vi "Dark Current Test All Files For Experiments.vi"() -> ()   [LabVIEW 2020]
uses:
  <instrlib>/CAEN PSM/CAEN PSM.lvlib
panel:
  out "Test is Running 2":bool
  in  "Begin Test 2":bool
  out "7 2":bool
  out "6 2":bool
  out "8 2":bool
  out "5 2":bool
  out "4 2":bool
  out "3 2":bool
  out "2 2":bool
  out "1 2":bool
  out "OVV? 4":bool=TRUE
  out "OVC? 4":bool=TRUE
  out "Actual Voltage Level (V) 4":dbl format="%#_13g"
  out "Actual Current Limit (nA) 2":dbl format="%#_13g"
  in  "dt (s) 2":i32
  out "Time Left (s) 2":dbl
  out "Power Supply Trip 2":bool
  in  "VISA resource name 3":refnum<visa-resource-name>
  in  "Channel # 2":i32
  out "Manual Measurments \nNeeded 2":bool
  in  "Barcodes 2":string[](array[string])
  out "OVV? 3":bool=TRUE
  out "OVC? 3":bool=TRUE
  out "Actual Voltage Level (V) 3":dbl format="%#_13g"
  out "Recorded Current\nfor Previous Tube 2":dbl format="%#_13g"
  in  "Measure Next Tube 2":bool
  out "Next Measurment 2":string
  in  "N 2":i32
  in  "VISA resource name 2":refnum<visa-resource-name>
  in  "Channel #":i32
  out "Power Supply Trip":bool
  out "Time Left (s)":dbl
  out "8":bool
  out "7":bool
  out "6":bool
  out "5":bool
  out "4":bool
  out "3":bool
  out "2":bool
  out "1":bool
  out "Test is Running":bool
  in  "Begin Test":bool
  out "Manual Measurments \nNeeded":bool
  out "OVV? 2":bool=TRUE
  out "OVC? 2":bool=TRUE
  out "Actual Voltage Level (V) 2":dbl format="%#_13g"
  out "Recorded Current\nfor Previous Tube":dbl format="%#_13g"
  in  "Measure Next Tube":bool
  in  "Barcodes":string[](array[string])
  out "Next Measurment":string
  in  "N":i32
  in  "dt (s)":i32
  out "Actual Current Limit (nA)":dbl format="%#_13g"
  out "Actual Voltage Level (V)":dbl format="%#_13g"
  out "OVC?":bool=TRUE
  out "OVV?":bool=TRUE
  # "Dark Current Test"
  # "Instructions in Brief:\n1. Begin the program by clicking the white arrow.\n2. Assemble tubes into the test bench.\n3. Select COM5 for the \"VISA resource name\".\n4. Enter in how often you want to take measurement in the \"dt\" box (typically 60s)\n5. Enter in how many measurments you want to take (typically 15)\n6. Scan in the 8 tubes that you are testing.\n(If you take 15 measurments every 60s, the test will take 15 min.)\n7. Click \"Begin Test\". The \"Test is Running\" LED should light up.\n8. After the intial test, if the total current is below 16nA, \n    the program will write the \n     file and end the test.\n9. If the total current is above 16nA, manual\n    measurments need to be taken.\n10. Engage only the tube indicated by \"Next Measurment\". \n11. Click \"Measure\".\n12. Engage the next tube and continue untill all have been measured.\n13. In both cases, the program will write files and end the test. \n14. The test is over when the \"Test is Running\" LED has turned off."
  # "Green lights indicate tubes that have passed."
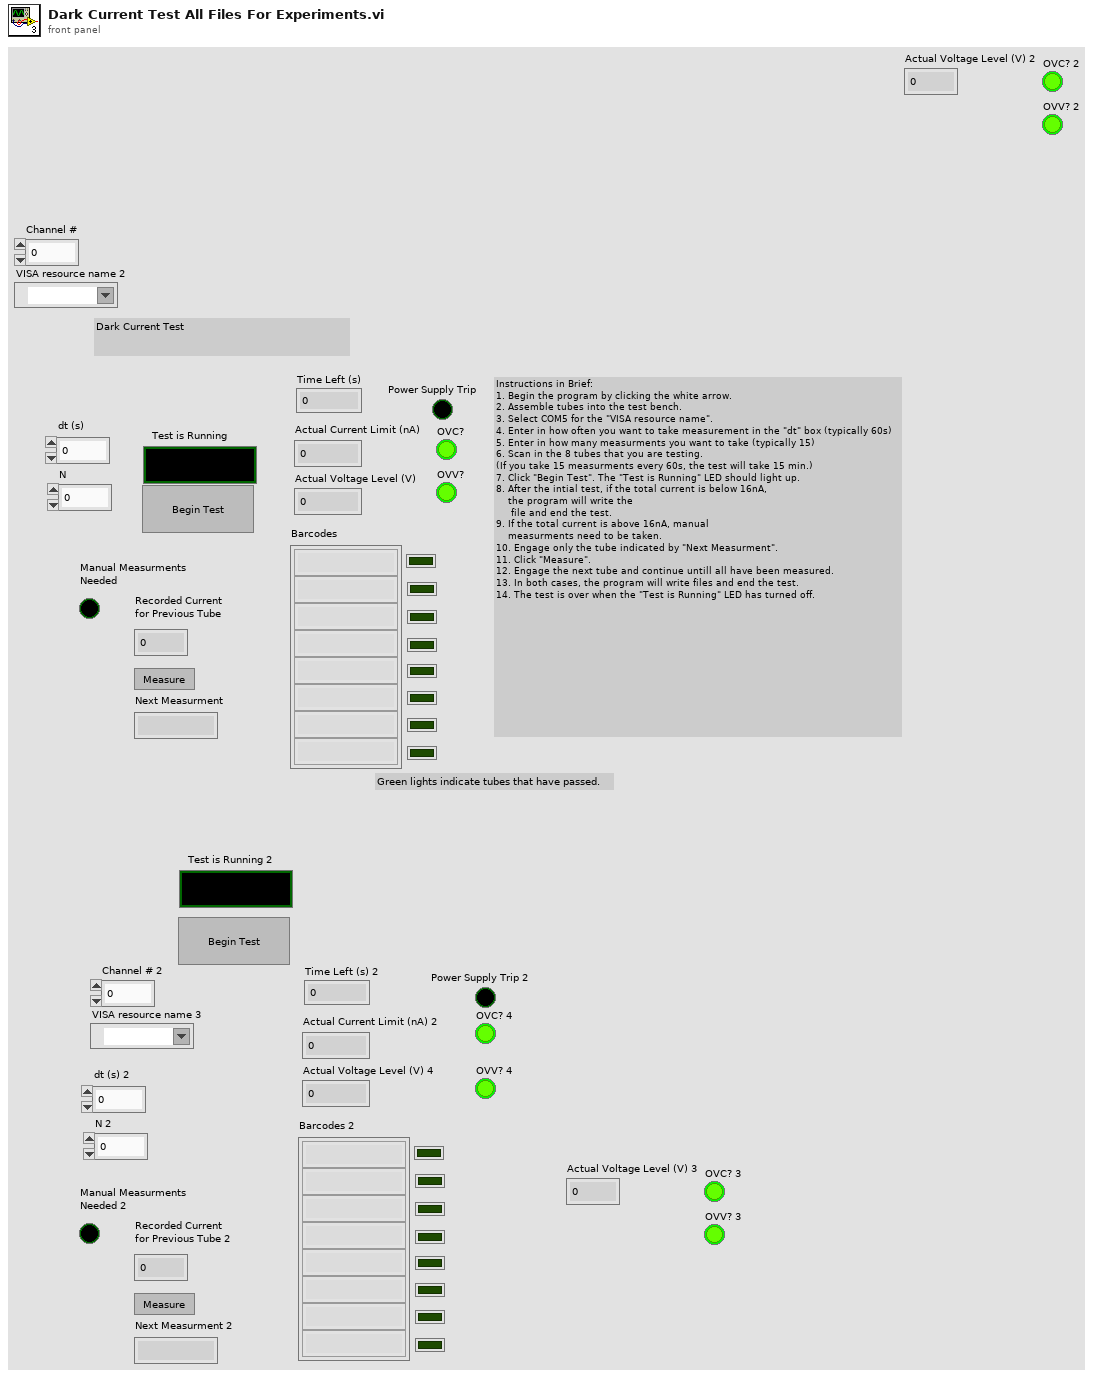
[diagram p1: front panel]
types:
  T1 = cluster{"VISA resource name":refnum<visa-resource-name>, "Board address":u8, "NChannels":u8}
  T2 = cluster{"ON":bool, "RUP":bool, "RDW":bool, "OVC":bool, "OVV":bool, "UNV":bool, "MAXV":bool, "TRIP":bool, "OVP":bool, "OVT":bool, "DIS":bool, "KILL":bool, "ILK":bool, "NOCAL":bool}[]
  T3 = cluster{"ON":bool, "RUP":bool, "RDW":bool, "OVC":bool, "OVV":bool, "UNV":bool, "MAXV":bool, "TRIP":bool, "OVP":bool, "OVT":bool, "DIS":bool, "KILL":bool, "ILK":bool, "NOCAL":bool}
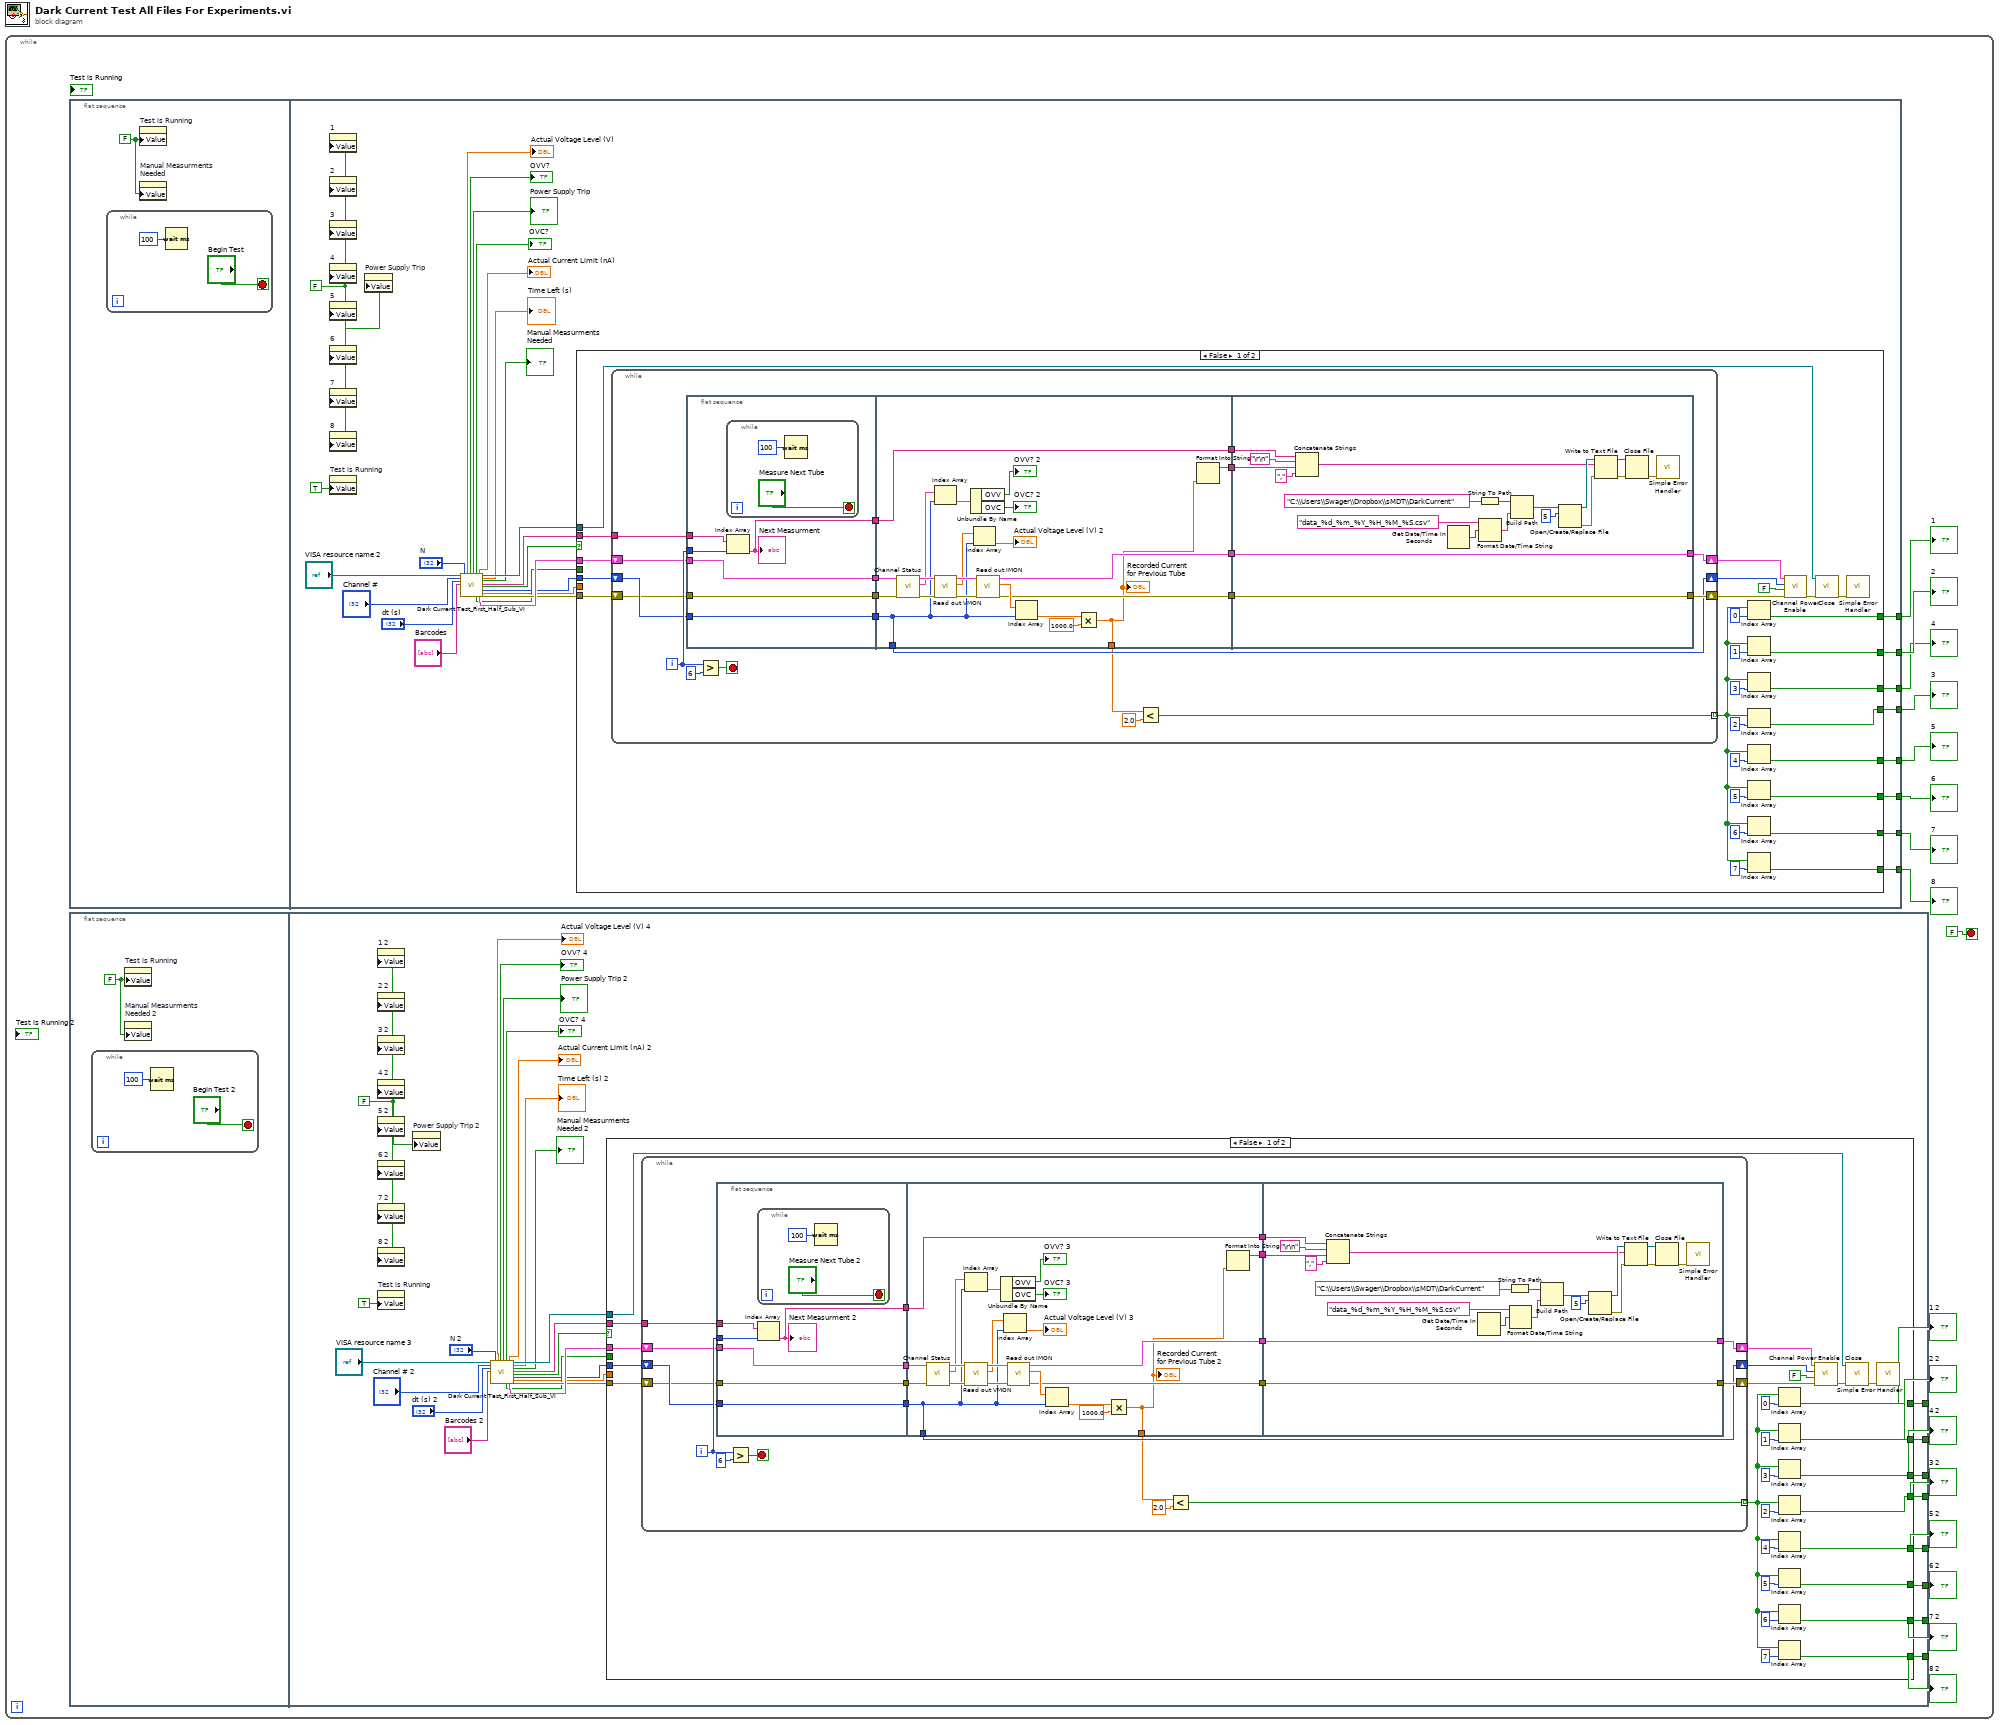
[diagram p0: block diagram]
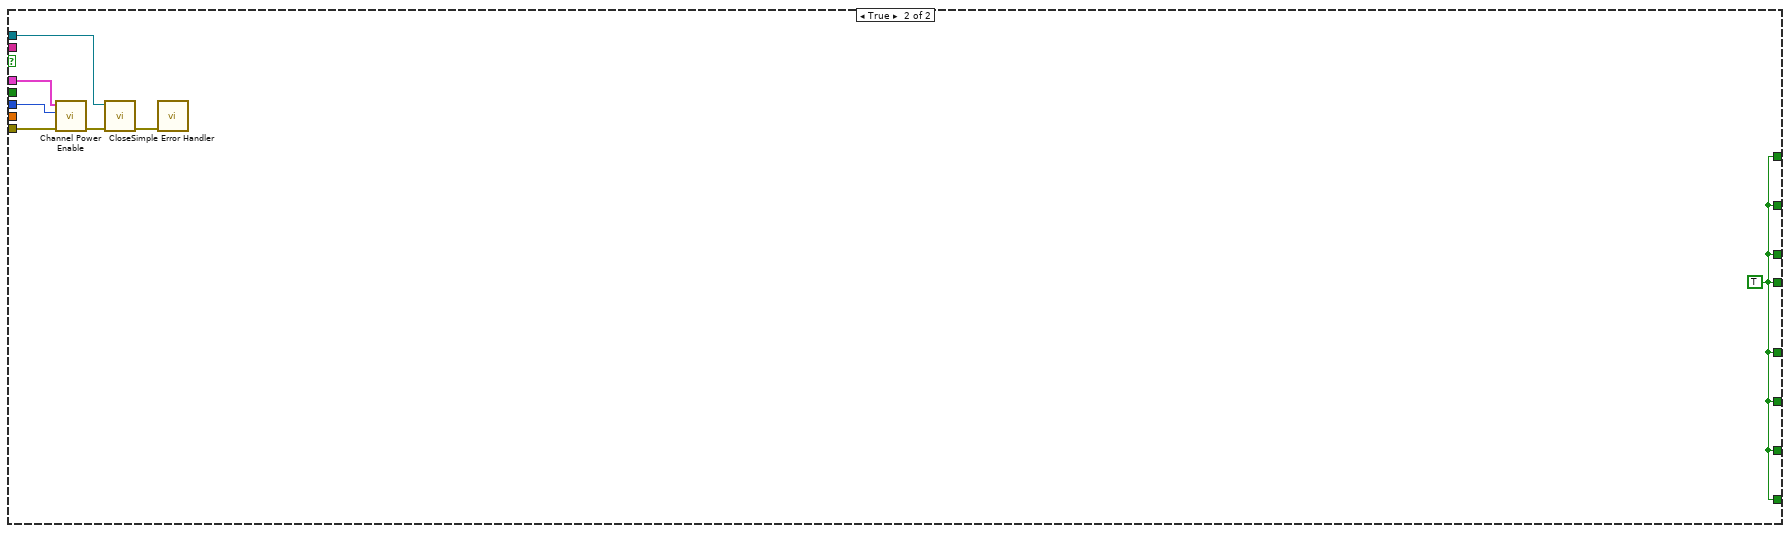
[diagram p2: hidden frame]
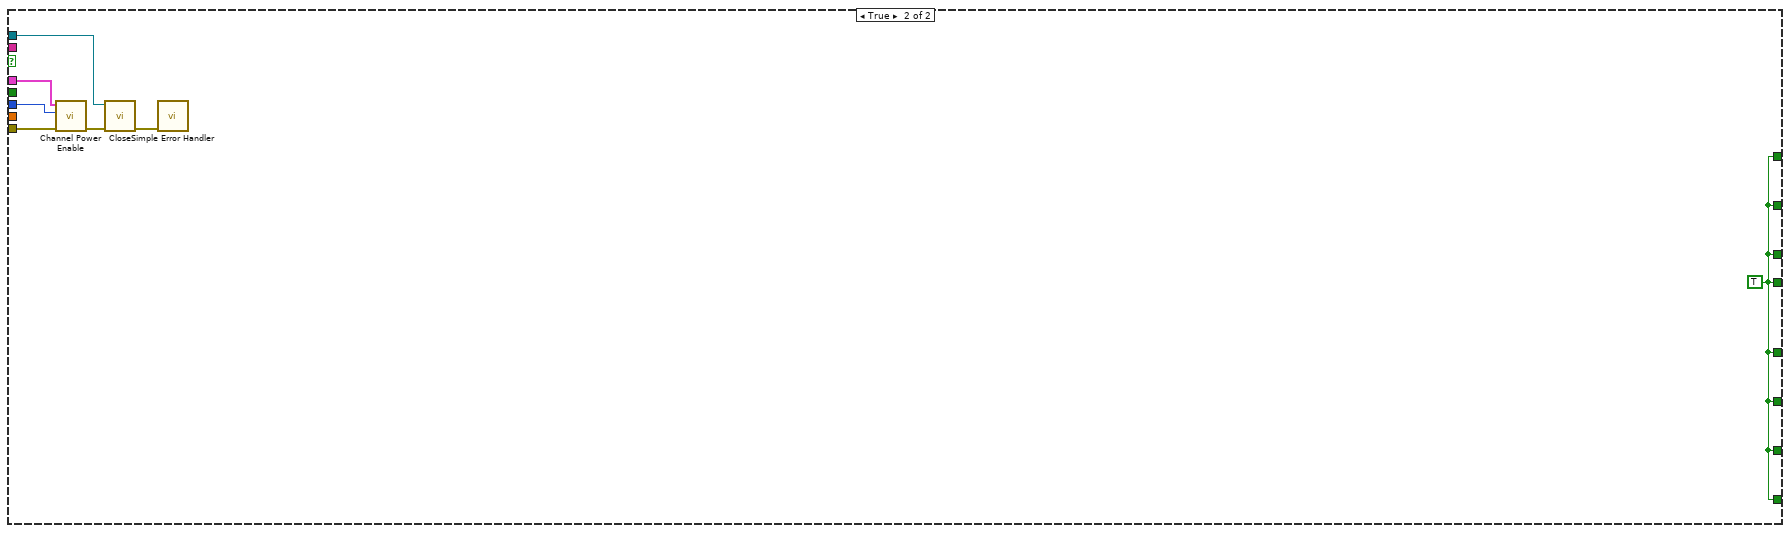
[diagram p3: hidden frame]
diagram:
  n1 = while {
    stop <- FALSE stop-if-true
    n2 = flat-sequence {
      tunnel: [w181] -> w16
      tunnel: [w180] -> w15
      tunnel: [w179] -> w14
      tunnel: [w178] -> w13
      tunnel: [w177] -> w12
      tunnel: [w176] -> w11
      tunnel: [w175] -> w10
      tunnel: [w174] -> w9
      frame #0 {
        w155 = FALSE
        n3 = while {
          stop <- "Begin Test" stop-if-true
          n4 = Wait (ms)(milliseconds to wait=100) -> ()  [unwired: 1 out]
        }
        n5 = property on="Test is Running" class="Bool (strict)"("Value"=w155) -> ()  [unwired: 2 in, 2 out]
        n6 = property on="Manual Measurments \nNeeded" class="Bool (strict)"("Value"=w155) -> ()  [unwired: 2 in, 2 out]
      }
      frame #1 {
        w159 = FALSE
        n7 = property on="1" class="Bool (strict)"("Value"=w159) -> ()  [unwired: 2 in, 2 out]
        n8 = property on="2" class="Bool (strict)"("Value"=w159) -> ()  [unwired: 2 in, 2 out]
        n9 = property on="3" class="Bool (strict)"("Value"=w159) -> ()  [unwired: 2 in, 2 out]
        n10 = property on="4" class="Bool (strict)"("Value"=w159) -> ()  [unwired: 2 in, 2 out]
        n11 = property on="5" class="Bool (strict)"("Value"=w159) -> ()  [unwired: 2 in, 2 out]
        n12 = property on="6" class="Bool (strict)"("Value"=w159) -> ()  [unwired: 2 in, 2 out]
        n13 = property on="7" class="Bool (strict)"("Value"=w159) -> ()  [unwired: 2 in, 2 out]
        n14 = property on="8" class="Bool (strict)"("Value"=w159) -> ()  [unwired: 2 in, 2 out]
        n15 = property on="Test is Running" class="Bool (strict)"("Value"=TRUE) -> ()  [unwired: 2 in, 2 out]
        n16 = property on="Power Supply Trip" class="Bool (strict)"("Value"=w159) -> ()  [unwired: 2 in, 2 out]
        n17 = call "Dark Current Test_First_Half_Sub_VI.vi"("VISA Refnum in"="VISA resource name 2", "Channel #"="Channel #", "dt (s)"="dt (s)", "Barcodes in"="Barcodes", "N"="N") -> ("Actual Voltage Level (V)"=→"Actual Voltage Level (V)":dbl, "OVV?"=→"OVV?":bool, "Power Supply Trip"=→"Power Supply Trip":bool, "OVC?"=→"OVC?":bool, "Boolean 2"=w184:bool, "Actual Current Limit (nA)"=→"Actual Current Limit (nA)":dbl, "BoardHandle out 2"=w186:T1, "VISA Refnum out"=w170:refnum<visa-resource-name>, "Time Left (s)"=→"Time Left (s)":dbl, "Manual Measurments \nNeeded"=→"Manual Measurments \nNeeded":bool, "Barcodes out"=w172:string[], "Boolean"=w182:bool, "Channel # 3"=w183:i32, "Array"=w173:dbl[], "error out"=w185:errorcluster)  [unwired: 8 in]
        n18 = case shown="False" w182 {
          tunnel: w186 -> [w214 w287]
          tunnel: w185 -> [w215 w286]
          tunnel: w184 -> [_ _]
          tunnel: w183 -> [w213 w285]
          tunnel: w170 -> [w209 w288]
          tunnel: w173 -> [_ _]
          tunnel: w172 -> [w205 _]
          tunnel: [w195 w291] -> w181
          tunnel: [w194 w291] -> w180
          tunnel: [w193 w291] -> w179
          tunnel: [w192 w291] -> w178
          tunnel: [w191 w291] -> w177
          tunnel: [w190 w291] -> w176
          tunnel: [w189 w291] -> w175
          tunnel: [w188 w291] -> w174
          frame False {
            n19 = while {
              shift-right: [w221] -> w206
              shift-left: w213 -> [w231]
              shift-right: [w223] -> w208
              shift-left: w214 -> [w228]
              shift-right: [w222] -> w207
              shift-left: w215 -> [w226]
              tunnel: w205 -> [w219]
              tunnel: [w216] -> w204 mode=indexing
              i -> [w234]
              stop <- w235 stop-if-true
              n20 = flat-sequence {
                tunnel: w234 -> [w242]
                tunnel: [w241] -> w233
                tunnel: w231 -> [w240]
                tunnel: [w240] -> w230
                tunnel: [w239] -> w229
                tunnel: w228 -> [w239]
                tunnel: [w238] -> w227
                tunnel: w226 -> [w238]
                tunnel: w219 -> [w237]
                tunnel: w233 -> [w252]
                tunnel: [w252] -> w232
                tunnel: w230 -> [w247]
                tunnel: w229 -> [w250]
                tunnel: w227 -> [w251]
                tunnel: [w249] -> w225
                tunnel: [w248] -> w224
                tunnel: [w247] -> w221
                tunnel: [w246] -> w220
                tunnel: [w245] -> w218
                tunnel: w232 -> [w270]
                tunnel: w225 -> [w268]
                tunnel: w224 -> [w267]
                tunnel: [w268] -> w223
                tunnel: [w267] -> w222
                tunnel: w220 -> [w266]
                frame #0 {
                  n21 = while {
                    stop <- "Measure Next Tube" stop-if-true
                    n22 = Wait (ms)(milliseconds to wait=100) -> ()  [unwired: 1 out]
                  }
                  n23 = Index Array(array=w237, index=w242) -> (element=w241:string)
                  "Next Measurment" <- w241
                }
                frame #1 {
                  n24 = call <instrlib>:"Channel Status.vi"("error in (no error)"=w251, "BoardHandle"=w250) -> ("error out"=w258:errorcluster, "Channel Status Array"=w254:T2, "BoardHandle out"=w259:T1)  [unwired: 7 in]
                  n25 = Index Array(array=w254, index=w247) -> (element=w255:T3)
                  n26 = call <instrlib>:"Read out VMON.vi"("error in (no error)"=w258, "BoardHandle"=w259) -> ("error out"=w262:errorcluster, "VMon values (V)"=w260:dbl[], "BoardHandle out"=w261:T1)  [unwired: 7 in]
                  n27 = Unbundle By Name(w255) -> ("OVV"=→"OVV? 2":bool, "OVC"=→"OVC? 2":bool)
                  n28 = Index Array(array=w260, index=w247) -> (element=→"Actual Voltage Level (V) 2":dbl)
                  n29 = call <instrlib>:"Read out IMON.vi"("error in (no error)"=w262, "BoardHandle"=w261) -> ("error out"=w248:errorcluster, "IMon values (uA)"=w265:dbl[], "BoardHandle out"=w249:T1)  [unwired: 6 in, 1 out]
                  n30 = Index Array(array=w265, index=w247) -> (element=w263:dbl)
                  n31 = Multiply(x=w263, y=1000.0) -> (x*y=w245:dbl)
                  "Recorded Current\nfor Previous Tube" <- w245
                  n32 = Format Into String(w245) -> (resulting string=w246:string)  [unwired: 3 in, 1 out]
                }
                frame #2 {
                  n33 = Concatenate Strings(w270, "\r\n", w266, ",") -> (w272:string)
                  n34 = Get Date/Time In Seconds() -> (seconds since 1Jan1904=w282:timestamp)
                  n35 = String To Path(string="C:\\Users\\Swager\\Dropbox\\sMDT\\DarkCurrent") -> (path=w281:path)
                  n36 = Format Date/Time String(time format string (%c)="data_%d_%m_%Y_%H_%M_%S.csv", seconds (now)=w282) -> (date/time string=w283:string)  [unwired: 1 in]
                  n37 = Build Path(base path=w281, name or relative path=w283) -> (appended path=w279:path)
                  n38 = Open/Create/Replace File(file path (use dialog)=w279, operation (0:open)=5) -> (refnum out=w278:refnum<file>, error out=w277:errorcluster)  [unwired: 4 in, 1 out]
                  n39 = Write to Text File(file (use dialog)=w278, text=w272, error in=w277) -> (refnum out=w276:refnum<file>, error out=w275:errorcluster)  [unwired: 1 in, 1 out]
                  n40 = Close File(refnum=w276, error in=w275) -> (error out=w274:errorcluster)  [unwired: 1 out]
                  n41 = call <vilib>:"Simple Error Handler.vi"("error in (no error)"=w274) -> ()  [unwired: 4 in, 5 out]
                }
              }
              n42 = Greater?(x=w234, y=6) -> (0:w235:bool)
              n43 = Less?(x=w218, y=2.0) -> (x < y?=w216:bool)
            }
            n44 = Index Array(array=w204, index=0) -> (element=w195:bool)
            n45 = Index Array(array=w204, index=1) -> (element=w194:bool)
            n46 = Index Array(array=w204, index=3) -> (element=w192:bool)
            n47 = Index Array(array=w204, index=2) -> (element=w193:bool)
            n48 = Index Array(array=w204, index=4) -> (element=w191:bool)
            n49 = Index Array(array=w204, index=5) -> (element=w190:bool)
            n50 = Index Array(array=w204, index=6) -> (element=w189:bool)
            n51 = Index Array(array=w204, index=7) -> (element=w188:bool)
            n52 = call <instrlib>:"Channel Power Enable.vi"("error in (no error)"=w207, "Enable (OFF)"=FALSE, "Channel (0)"=w206, "BoardHandle"=w208) -> ("error out"=w211:errorcluster)  [unwired: 6 in, 1 out]
            n53 = call <instrlib>:"Close.vi"("error in (no error)"=w211, "VISA resource name"=w209) -> ("error out"=w210:errorcluster)  [unwired: 9 in]
            n54 = call <vilib>:"Simple Error Handler.vi"("error in (no error)"=w210) -> ()  [unwired: 4 in, 5 out]
          }
          frame True {
            w291 = TRUE
            n55 = call <instrlib>:"Channel Power Enable.vi"("error in (no error)"=w286, "Channel (0)"=w285, "BoardHandle"=w287) -> ("error out"=w290:errorcluster)  [unwired: 7 in, 1 out]
            n56 = call <instrlib>:"Close.vi"("error in (no error)"=w290, "VISA resource name"=w288) -> ("error out"=w289:errorcluster)  [unwired: 9 in]
            n57 = call <vilib>:"Simple Error Handler.vi"("error in (no error)"=w289) -> ()  [unwired: 4 in, 5 out]
          }
        }
      }
    }
    n58 = flat-sequence {
      tunnel: [w30] -> w8
      tunnel: [w29] -> w7
      tunnel: [w28] -> w6
      tunnel: [w27] -> w5
      tunnel: [w26] -> w4
      tunnel: [w25] -> w3
      tunnel: [w24] -> w2
      tunnel: [w23] -> w1
      frame #0 {
        w18 = FALSE
        n59 = while {
          stop <- "Begin Test 2" stop-if-true
          n60 = Wait (ms)(milliseconds to wait=100) -> ()  [unwired: 1 out]
        }
        n61 = property on="Test is Running" class="Bool (strict)"("Value"=w18) -> ()  [unwired: 2 in, 2 out]
        n62 = property on="Manual Measurments \nNeeded 2" class="Bool (strict)"("Value"=w18) -> ()  [unwired: 2 in, 2 out]
      }
      frame #1 {
        w22 = FALSE
        n63 = property on="1 2" class="Bool (strict)"("Value"=w22) -> ()  [unwired: 2 in, 2 out]
        n64 = property on="2 2" class="Bool (strict)"("Value"=w22) -> ()  [unwired: 2 in, 2 out]
        n65 = property on="3 2" class="Bool (strict)"("Value"=w22) -> ()  [unwired: 2 in, 2 out]
        n66 = property on="4 2" class="Bool (strict)"("Value"=w22) -> ()  [unwired: 2 in, 2 out]
        n67 = property on="5 2" class="Bool (strict)"("Value"=w22) -> ()  [unwired: 2 in, 2 out]
        n68 = property on="6 2" class="Bool (strict)"("Value"=w22) -> ()  [unwired: 2 in, 2 out]
        n69 = property on="7 2" class="Bool (strict)"("Value"=w22) -> ()  [unwired: 2 in, 2 out]
        n70 = property on="8 2" class="Bool (strict)"("Value"=w22) -> ()  [unwired: 2 in, 2 out]
        n71 = property on="Test is Running" class="Bool (strict)"("Value"=TRUE) -> ()  [unwired: 2 in, 2 out]
        n72 = property on="Power Supply Trip 2" class="Bool (strict)"("Value"=w22) -> ()  [unwired: 2 in, 2 out]
        n73 = call "Dark Current Test_First_Half_Sub_VI.vi"("VISA Refnum in"="VISA resource name 3", "Channel #"="Channel # 2", "dt (s)"="dt (s) 2", "Barcodes in"="Barcodes 2", "N"="N 2") -> ("Actual Voltage Level (V)"=→"Actual Voltage Level (V) 4":dbl, "OVV?"=→"OVV? 4":bool, "Power Supply Trip"=→"Power Supply Trip 2":bool, "OVC?"=→"OVC? 4":bool, "Boolean 2"=w47:bool, "Actual Current Limit (nA)"=→"Actual Current Limit (nA) 2":dbl, "BoardHandle out 2"=w49:T1, "VISA Refnum out"=w41:refnum<visa-resource-name>, "Time Left (s)"=→"Time Left (s) 2":dbl, "Manual Measurments \nNeeded"=→"Manual Measurments \nNeeded 2":bool, "Barcodes out"=w43:string[], "Boolean"=w45:bool, "Channel # 3"=w46:i32, "Array"=w44:dbl[], "error out"=w48:errorcluster)  [unwired: 8 in]
        n74 = case shown="False" w45 {
          tunnel: w49 -> [w77 w150]
          tunnel: w48 -> [w78 w149]
          tunnel: w47 -> [_ _]
          tunnel: w46 -> [w76 w148]
          tunnel: w41 -> [w72 w151]
          tunnel: w44 -> [_ _]
          tunnel: w43 -> [w68 _]
          tunnel: [w58 w154] -> w23
          tunnel: [w57 w154] -> w24
          tunnel: [w56 w154] -> w26
          tunnel: [w55 w154] -> w25
          tunnel: [w54 w154] -> w27
          tunnel: [w53 w154] -> w28
          tunnel: [w52 w154] -> w29
          tunnel: [w51 w154] -> w30
          frame False {
            n75 = while {
              shift-right: [w84] -> w69
              shift-left: w76 -> [w94]
              shift-right: [w86] -> w71
              shift-left: w77 -> [w91]
              shift-right: [w85] -> w70
              shift-left: w78 -> [w89]
              tunnel: w68 -> [w82]
              tunnel: [w79] -> w67 mode=indexing
              i -> [w97]
              stop <- w98 stop-if-true
              n76 = flat-sequence {
                tunnel: w97 -> [w105]
                tunnel: [w104] -> w96
                tunnel: w94 -> [w103]
                tunnel: [w103] -> w93
                tunnel: [w102] -> w92
                tunnel: w91 -> [w102]
                tunnel: [w101] -> w90
                tunnel: w89 -> [w101]
                tunnel: w82 -> [w100]
                tunnel: w96 -> [w115]
                tunnel: [w115] -> w95
                tunnel: w93 -> [w110]
                tunnel: w92 -> [w113]
                tunnel: w90 -> [w114]
                tunnel: [w112] -> w88
                tunnel: [w111] -> w87
                tunnel: [w110] -> w84
                tunnel: [w109] -> w83
                tunnel: [w108] -> w81
                tunnel: w95 -> [w133]
                tunnel: w88 -> [w131]
                tunnel: w87 -> [w130]
                tunnel: [w131] -> w86
                tunnel: [w130] -> w85
                tunnel: w83 -> [w129]
                frame #0 {
                  n77 = while {
                    stop <- "Measure Next Tube 2" stop-if-true
                    n78 = Wait (ms)(milliseconds to wait=100) -> ()  [unwired: 1 out]
                  }
                  n79 = Index Array(array=w100, index=w105) -> (element=w104:string)
                  "Next Measurment 2" <- w104
                }
                frame #1 {
                  n80 = call <instrlib>:"Channel Status.vi"("error in (no error)"=w114, "BoardHandle"=w113) -> ("error out"=w121:errorcluster, "Channel Status Array"=w117:T2, "BoardHandle out"=w122:T1)  [unwired: 7 in]
                  n81 = Index Array(array=w117, index=w110) -> (element=w118:T3)
                  n82 = call <instrlib>:"Read out VMON.vi"("error in (no error)"=w121, "BoardHandle"=w122) -> ("error out"=w125:errorcluster, "VMon values (V)"=w123:dbl[], "BoardHandle out"=w124:T1)  [unwired: 7 in]
                  n83 = Unbundle By Name(w118) -> ("OVV"=→"OVV? 3":bool, "OVC"=→"OVC? 3":bool)
                  n84 = Index Array(array=w123, index=w110) -> (element=→"Actual Voltage Level (V) 3":dbl)
                  n85 = call <instrlib>:"Read out IMON.vi"("error in (no error)"=w125, "BoardHandle"=w124) -> ("error out"=w111:errorcluster, "IMon values (uA)"=w128:dbl[], "BoardHandle out"=w112:T1)  [unwired: 6 in, 1 out]
                  n86 = Index Array(array=w128, index=w110) -> (element=w126:dbl)
                  n87 = Multiply(x=w126, y=1000.0) -> (x*y=w108:dbl)
                  "Recorded Current\nfor Previous Tube 2" <- w108
                  n88 = Format Into String(w108) -> (resulting string=w109:string)  [unwired: 3 in, 1 out]
                }
                frame #2 {
                  n89 = Concatenate Strings(w133, "\r\n", w129, ",") -> (w135:string)
                  n90 = Get Date/Time In Seconds() -> (seconds since 1Jan1904=w145:timestamp)
                  n91 = String To Path(string="C:\\Users\\Swager\\Dropbox\\sMDT\\DarkCurrent") -> (path=w144:path)
                  n92 = Format Date/Time String(time format string (%c)="data_%d_%m_%Y_%H_%M_%S.csv", seconds (now)=w145) -> (date/time string=w146:string)  [unwired: 1 in]
                  n93 = Build Path(base path=w144, name or relative path=w146) -> (appended path=w142:path)
                  n94 = Open/Create/Replace File(file path (use dialog)=w142, operation (0:open)=5) -> (refnum out=w141:refnum<file>, error out=w140:errorcluster)  [unwired: 4 in, 1 out]
                  n95 = Write to Text File(file (use dialog)=w141, text=w135, error in=w140) -> (refnum out=w139:refnum<file>, error out=w138:errorcluster)  [unwired: 1 in, 1 out]
                  n96 = Close File(refnum=w139, error in=w138) -> (error out=w137:errorcluster)  [unwired: 1 out]
                  n97 = call <vilib>:"Simple Error Handler.vi"("error in (no error)"=w137) -> ()  [unwired: 4 in, 5 out]
                }
              }
              n98 = Greater?(x=w97, y=6) -> (0:w98:bool)
              n99 = Less?(x=w81, y=2.0) -> (x < y?=w79:bool)
            }
            n100 = Index Array(array=w67, index=0) -> (element=w58:bool)
            n101 = Index Array(array=w67, index=1) -> (element=w57:bool)
            n102 = Index Array(array=w67, index=3) -> (element=w55:bool)
            n103 = Index Array(array=w67, index=2) -> (element=w56:bool)
            n104 = Index Array(array=w67, index=4) -> (element=w54:bool)
            n105 = Index Array(array=w67, index=5) -> (element=w53:bool)
            n106 = Index Array(array=w67, index=6) -> (element=w52:bool)
            n107 = Index Array(array=w67, index=7) -> (element=w51:bool)
            n108 = call <instrlib>:"Channel Power Enable.vi"("error in (no error)"=w70, "Enable (OFF)"=FALSE, "Channel (0)"=w69, "BoardHandle"=w71) -> ("error out"=w74:errorcluster)  [unwired: 6 in, 1 out]
            n109 = call <instrlib>:"Close.vi"("error in (no error)"=w74, "VISA resource name"=w72) -> ("error out"=w73:errorcluster)  [unwired: 9 in]
            n110 = call <vilib>:"Simple Error Handler.vi"("error in (no error)"=w73) -> ()  [unwired: 4 in, 5 out]
          }
          frame True {
            w154 = TRUE
            n111 = call <instrlib>:"Channel Power Enable.vi"("error in (no error)"=w149, "Channel (0)"=w148, "BoardHandle"=w150) -> ("error out"=w153:errorcluster)  [unwired: 7 in, 1 out]
            n112 = call <instrlib>:"Close.vi"("error in (no error)"=w153, "VISA resource name"=w151) -> ("error out"=w152:errorcluster)  [unwired: 9 in]
            n113 = call <vilib>:"Simple Error Handler.vi"("error in (no error)"=w152) -> ()  [unwired: 4 in, 5 out]
          }
        }
      }
    }
    "1" <- w16
    "2" <- w15
    "3" <- w14
    "4" <- w13
    "5" <- w12
    "8" <- w9
    "6" <- w11
    "7" <- w10
    "1 2" <- w1
    "2 2" <- w2
    "3 2" <- w4
    "4 2" <- w3
    "5 2" <- w5
    "8 2" <- w8
    "6 2" <- w6
    "7 2" <- w7
  }
